vi "CheexyDrive_handledeadband.vi"(10 "Deadband":dbl, 11 "val":dbl) -> (3 "Val Out":dbl)   [LabVIEW 2016]
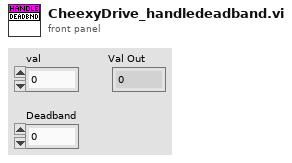
[diagram p1: front panel]
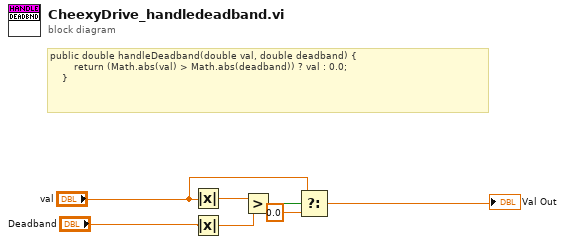
[diagram p0: block diagram]
diagram:
  # "public double handleDeadband(double val, double deadband) {\n        return (Math.abs(val) > Math.abs(deadband)) ? val : 0.0;\n    }"
  n1 = Absolute Value(x="val") -> (abs(x)=w4:dbl)
  n2 = Absolute Value(x="Deadband") -> (abs(x)=w3:dbl)
  n3 = Greater?(x=w4, y=w3) -> (0:w2:bool)
  n4 = Select(t="val", s=w2, f=0.0) -> (s? t:f=→"Val Out":dbl)
